vi "Initialize.vi"(8 "error in (no error)":errorcluster, 9 "Reset? (T: Yes)":bool=TRUE, 10 "ID Query? (T: Yes)":bool=TRUE, 11 "VISA resource name":refnum<visa-resource-name>) -> (0 "error out":errorcluster, 2 "Device info":T1, 3 "VISA resource name out":refnum<visa-resource-name>)   [LabVIEW 2012, in "Tektronix TTR500 Series.lvlib"]
doc: "Establishes communication with the instrument and optionally performs an instrument identification query and/or an instrument reset. It also places the instrument in a default state needed for other instrument driver operations. Therefore, call this VI before calling other instrument driver VIs for this instrument. Generally, you need to call the <B>Initialize VI</B> only once at the beginning of an application."
uses:
  <instrlib>/Tektronix TTR500 Series/Tektronix TTR500 Series.lvlib
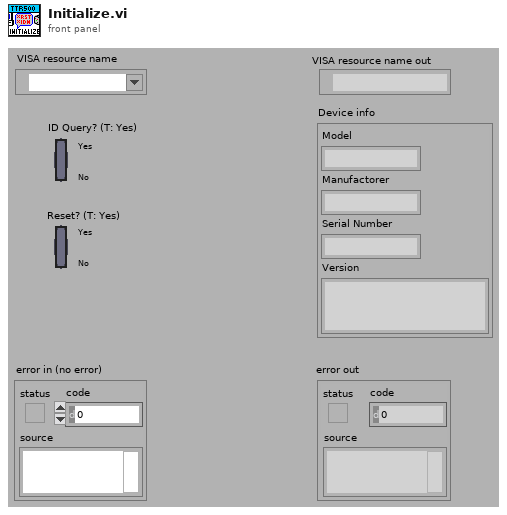
[diagram p1: front panel]
types:
  T1 = cluster{"Model":string, "Manufactorer":string, "Serial Number":string, "Version ":string}
  T2 = cluster{"Status":bool, "Code":i32, "Source (VI Name)":string}
  T3 = cluster{"[0]":string, "[1]":string, "[2]":string, "[3]":string}
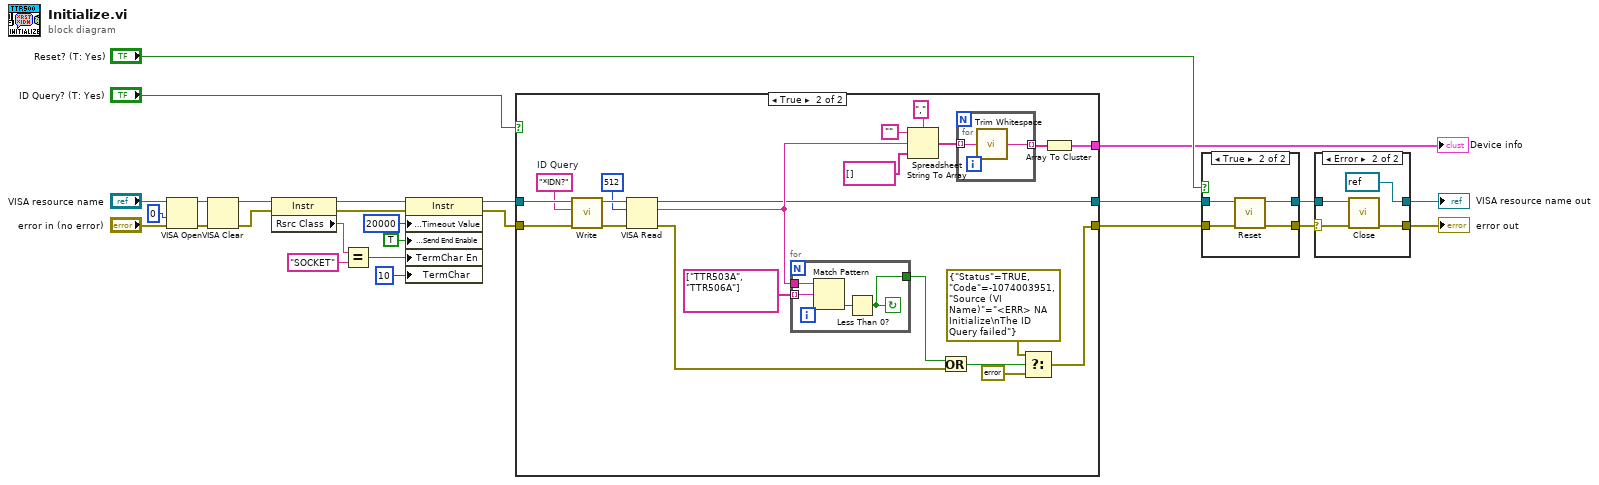
[diagram p0: block diagram]
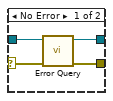
[diagram p2: hidden frame]
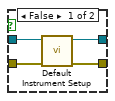
[diagram p3: hidden frame]
diagram:
  n1 = VISA Open(access mode=u32 0, error in (no error)="error in (no error)", VISA resource name="VISA resource name") -> (VISA resource name=w14:refnum<visa-resource-name>, error out=w15:errorcluster)  [unwired: 2 in]
  n2 = VISA Clear(VISA resource name=w14, error in (no error)=w15) -> (VISA resource name out=w4:refnum<visa-resource-name>, error out=w3:errorcluster)
  n3 = property class="Instr"(reference=w4, error in=w3) -> (reference out=w6:refnum<visa-resource-name>, error out=w5:errorcluster, "Rsrc Class"=w9:string)
  n4 = Equal?(x=w9, y="SOCKET") -> (x = y?=w7:bool)
  n5 = property class="Instr"(reference=w6, error in=w5, "General Settings:Timeout Value"=u32 20000, "Message Based Settings:Send End Enable"=TRUE, "TermChar En"=w7, "TermChar"=u8 10 ("Message Based Settings:Termination Character")) -> (reference out=w2:refnum<visa-resource-name>, error out=w1:errorcluster)
  n6 = case shown="True" "ID Query? (T: Yes)" {
    tunnel: [w27 w32] -> w25
    tunnel: [w28 w29] -> w26
    tunnel: w2 -> [w28 w48]
    tunnel: w1 -> [w27 w49]
    tunnel: [_ w30] -> w13
    frame False {
    }
    frame True {
      w44 = "*IDN?"  # ID Query
      n7 = call <instrlib>:"Write.vi"("error in (no error)"=w49, "String ()"=w44, "VISA resource name"=w48) -> ("error out"=w46:errorcluster, "VISA resource name out"=w47:refnum<visa-resource-name>)  [unwired: 6 in, 1 out]
      n8 = VISA Read(VISA resource name=w47, byte count=u32 512, error in (no error)=w46) -> (VISA resource name out=w29:refnum<visa-resource-name>, read buffer=w33:string, error out=w31:errorcluster)  [unwired: 1 out]
      n9 = for {
        tunnel: w33 -> [w53]
        tunnel: string[] ["TTR503A", "TTR506A"] ("string array") -> [w52] mode=indexing
        tunnel: [w50] -> w34
        stop <- w50 continue-if-true
        n10 = Match Pattern(string=w53, regular expression=w52) -> (offset past match=w51:i32)  [unwired: 1 in, 3 out]
        n11 = Less Than 0?(x=w51) -> (x < 0?=w50:bool)
      }
      n12 = Spreadsheet String To Array(delimiter (Tab)=",", format string="", spreadsheet string=w33, array type (2D Dbl)=string[] []) -> (array=w37:string[])
      n13 = Or(x=w34, y=w31) -> (x .or. y?=w43:bool)
      n14 = for {
        tunnel: w37 -> [w55] mode=indexing
        tunnel: [w54] -> w36 mode=indexing
        n15 = call <vilib>:"Trim Whitespace.vi"("string"=w55) -> ("trimmed string"=w54:string)  [unwired: 1 in]
      }
      n16 = Select(t=T2 {"Status"=TRUE, "Code"=-1074003951, "Source (VI Name)"="<ERR> NA Initialize\nThe ID Query failed"}, s=w43, f=T2 {"Status"=FALSE, "Code"=0, "Source (VI Name)"=""} ("t")) -> (s? t:f=w32:T2)
      n17 = Array To Cluster(array=w36) -> (cluster=w30:T3)
    }
  }
  "Device info" <- w13
  n18 = case shown="True" "Reset? (T: Yes)" {
    tunnel: w25 -> [w58 w60]
    tunnel: [w57 w63] -> w16
    tunnel: w26 -> [w59 w61]
    tunnel: [w56 w62] -> w17
    frame False {
      n19 = call <instrlib>:"Default Instrument Setup.vi"("error in (no error)"=w58, "VISA resource name"=w59) -> ("error out"=w57:errorcluster, "VISA resource name out"=w56:refnum<visa-resource-name>)  [unwired: 8 in]
    }
    frame True {
      n20 = call <instrlib>:"Reset.vi"("error in (no error)"=w60, "VISA resource name"=w61) -> ("error out"=w63:errorcluster, "VISA resource name out"=w62:refnum<visa-resource-name>)  [unwired: 8 in]
    }
  }
  n21 = case shown="Error" w16 {
    selector: w16 -> [w65 w69]
    tunnel: w17 -> [w64 w70]
    tunnel: [w67 refnum<visa-resource-name> refnum ("VISA resource name out")] -> w19
    tunnel: [w66 w71] -> w18
    frame No Error {
      n22 = call <instrlib>:"Error Query.vi"("error in (no error)"=w65, "VISA resource name"=w64) -> ("error out"=w66:errorcluster, "VISA resource name out"=w67:refnum<visa-resource-name>)  [unwired: 6 in, 2 out]
    }
    frame Error {
      n23 = call <instrlib>:"Close.vi"("error in (no error)"=w69, "VISA resource name"=w70) -> ("error out"=w71:errorcluster)  [unwired: 9 in]
    }
  }
  "VISA resource name out" <- w19
  "error out" <- w18
